vi "Sequence.Test.Engine.vi"(8 "error in (no error)":errorcluster, 11 "Data in":T1={"BeginTS"=timestamp(0 s since 1904-01-01), "EndTS"=timestamp(0 s since 1904-01-01), "State"=enum."Init", "Status.Work"=enum."-", "Status.Process"=enum."-", "Status.Home"=enum."-", "Status.Wabco"=enum."-", "Status.Client"=enum."-", "BreakReason"=enum."-", "BreakSource"=enum."-", "DoorLock"=FALSE, "Status.Prod"=[], "UserAction"={"Stop"=FALSE, "Pause"=FALSE, "Next"=FALSE}, "UserData"={"GuiMode"=enum."Process", "Test"={"IgnoreResults"=FALSE, "IgnoreImages"=FALSE, "ServiceMode"=FALSE}, "ContinueOrder"=FALSE}, "Error"={"status"=FALSE, "code"=0, "source"=""}, "Code"={"Ready"=FALSE, "DoubleOrder"=FALSE, "OrderDone"=FALSE, "AllowSingleSlot"=FALSE, "TunedA"=FALSE, "TunedB"=FALSE, "CheckDM"=FALSE, "ThresholdA"=0, "ThresholdB"=0, "Plate"=enum."Wabco", "ImgPath"=path "", "Variant"={"State"=enum."Init", "ImgPath"=path "", "WabcoPlate"="", "WabcoProduct"="", "ClientProduct"="", "ClientPlate"="", "TotalQuantity"=0, "OrderQuantity"=0, "Serial"=0, "Wabco"={"LaserJob"="", "AdditionalTxt"="037", "FactoryCode"="", "RevID"=0, "ForkID"=0, "FailuresLimit"=0, "GlobalCnt"=0, "Bank"=0, "SerialFormat"=enum."6 dig", "CoordA"={"X"=0.0, "Y"=0.0, "Angle"=0.0}, "CoordB"={"X"=0.0, "Y"=0.0, "Angle"=0.0}, "DMCconfig"=0}, "Client"={"LaserJob"="", "AdditionalTxt"="", "FactoryCode"="037", "RevID"=0, "ForkID"=0, "FailuresLimit"=0, "GlobalCnt"=0, "Bank"=0, "SerialFormat"=enum."6 dig", "CoordA"={"X"=0.0, "Y"=0.0, "Angle"=0.0}, "CoordB"={"X"=0.0, "Y"=0.0, "Angle"=0.0}, "DMCconfig"=0}}}, "Rotations"=0, "ProdIdx"=0, "ProdDone"=[], "PrintedSerials-Wabco"=[], "PrintedSerials-Client"=[], "Counters-Wabco"={"Expected"=0, "Done"=0, "OK"=0, "NOK"=0, "NOKlimit"=0, "Part"=0, "PartOK"=0}, "Counters-Client"={"Expected"=0, "Done"=0, "OK"=0, "NOK"=0, "NOKlimit"=0, "Part"=0, "PartOK"=0}}) -> (0 "error out":errorcluster, 3 "Data out":T1={"BeginTS"=timestamp(0 s since 1904-01-01), "EndTS"=timestamp(0 s since 1904-01-01), "State"=enum."Init", "Status.Work"=enum."-", "Status.Process"=enum."-", "Status.Home"=enum."-", "Status.Wabco"=enum."-", "Status.Client"=enum."-", "BreakReason"=enum."-", "BreakSource"=enum."-", "DoorLock"=FALSE, "Status.Prod"=[], "UserAction"={"Stop"=FALSE, "Pause"=FALSE, "Next"=FALSE}, "UserData"={"GuiMode"=enum."Process", "Test"={"IgnoreResults"=FALSE, "IgnoreImages"=FALSE, "ServiceMode"=FALSE}, "ContinueOrder"=FALSE}, "Error"={"status"=FALSE, "code"=0, "source"=""}, "Code"={"Ready"=FALSE, "DoubleOrder"=FALSE, "OrderDone"=FALSE, "AllowSingleSlot"=FALSE, "TunedA"=FALSE, "TunedB"=FALSE, "CheckDM"=FALSE, "ThresholdA"=0, "ThresholdB"=0, "Plate"=enum."Wabco", "ImgPath"=path "", "Variant"={"State"=enum."Init", "ImgPath"=path "", "WabcoPlate"="", "WabcoProduct"="", "ClientProduct"="", "ClientPlate"="", "TotalQuantity"=0, "OrderQuantity"=0, "Serial"=0, "Wabco"={"LaserJob"="", "AdditionalTxt"="037", "FactoryCode"="", "RevID"=0, "ForkID"=0, "FailuresLimit"=0, "GlobalCnt"=0, "Bank"=0, "SerialFormat"=enum."6 dig", "CoordA"={"X"=0.0, "Y"=0.0, "Angle"=0.0}, "CoordB"={"X"=0.0, "Y"=0.0, "Angle"=0.0}, "DMCconfig"=0}, "Client"={"LaserJob"="", "AdditionalTxt"="", "FactoryCode"="037", "RevID"=0, "ForkID"=0, "FailuresLimit"=0, "GlobalCnt"=0, "Bank"=0, "SerialFormat"=enum."6 dig", "CoordA"={"X"=0.0, "Y"=0.0, "Angle"=0.0}, "CoordB"={"X"=0.0, "Y"=0.0, "Angle"=0.0}, "DMCconfig"=0}}}, "Rotations"=0, "ProdIdx"=0, "ProdDone"=[], "PrintedSerials-Wabco"=[], "PrintedSerials-Client"=[], "Counters-Wabco"={"Expected"=0, "Done"=0, "OK"=0, "NOK"=0, "NOKlimit"=0, "Part"=0, "PartOK"=0}, "Counters-Client"={"Expected"=0, "Done"=0, "OK"=0, "NOK"=0, "NOKlimit"=0, "Part"=0, "PartOK"=0}})   [LabVIEW 2016]
uses:
  Sequence.Data.ctl
  Sequence.State.ctl
  Sequence.Step.Status.ctl
  Sequence.Test.BreakReason.ctl
  Sequence.Test.BreakSource.ctl
  Sequence.Test.Status.ctl
  Sequence.Slot.StatusData.ctl
  Sequence.Test.Unload.Status.ctl
  Sequence.Prod.StatusData.ctl
  Sequence.UserActions.ctl
  Sequence.UserData.ctl
  Sequence.MainMode.ctl
  Gui/MainGui.TestOptions.ctl
  Sequence.Code.Sets.ctl
  Sequence.PlateType.ctl
  Logger/Logger.Variant.Sets.ctl
  Station/Station.Changeover.State.vi
  Station/Station.Plate.Properties.ctl
  Sequence.Code.SerialFormat.ctl
  Drivers/V7310/LowLevel/V7310.Job.Sets.ctl
  Sequence.Counters.ctl
  Sequence.Global.vi
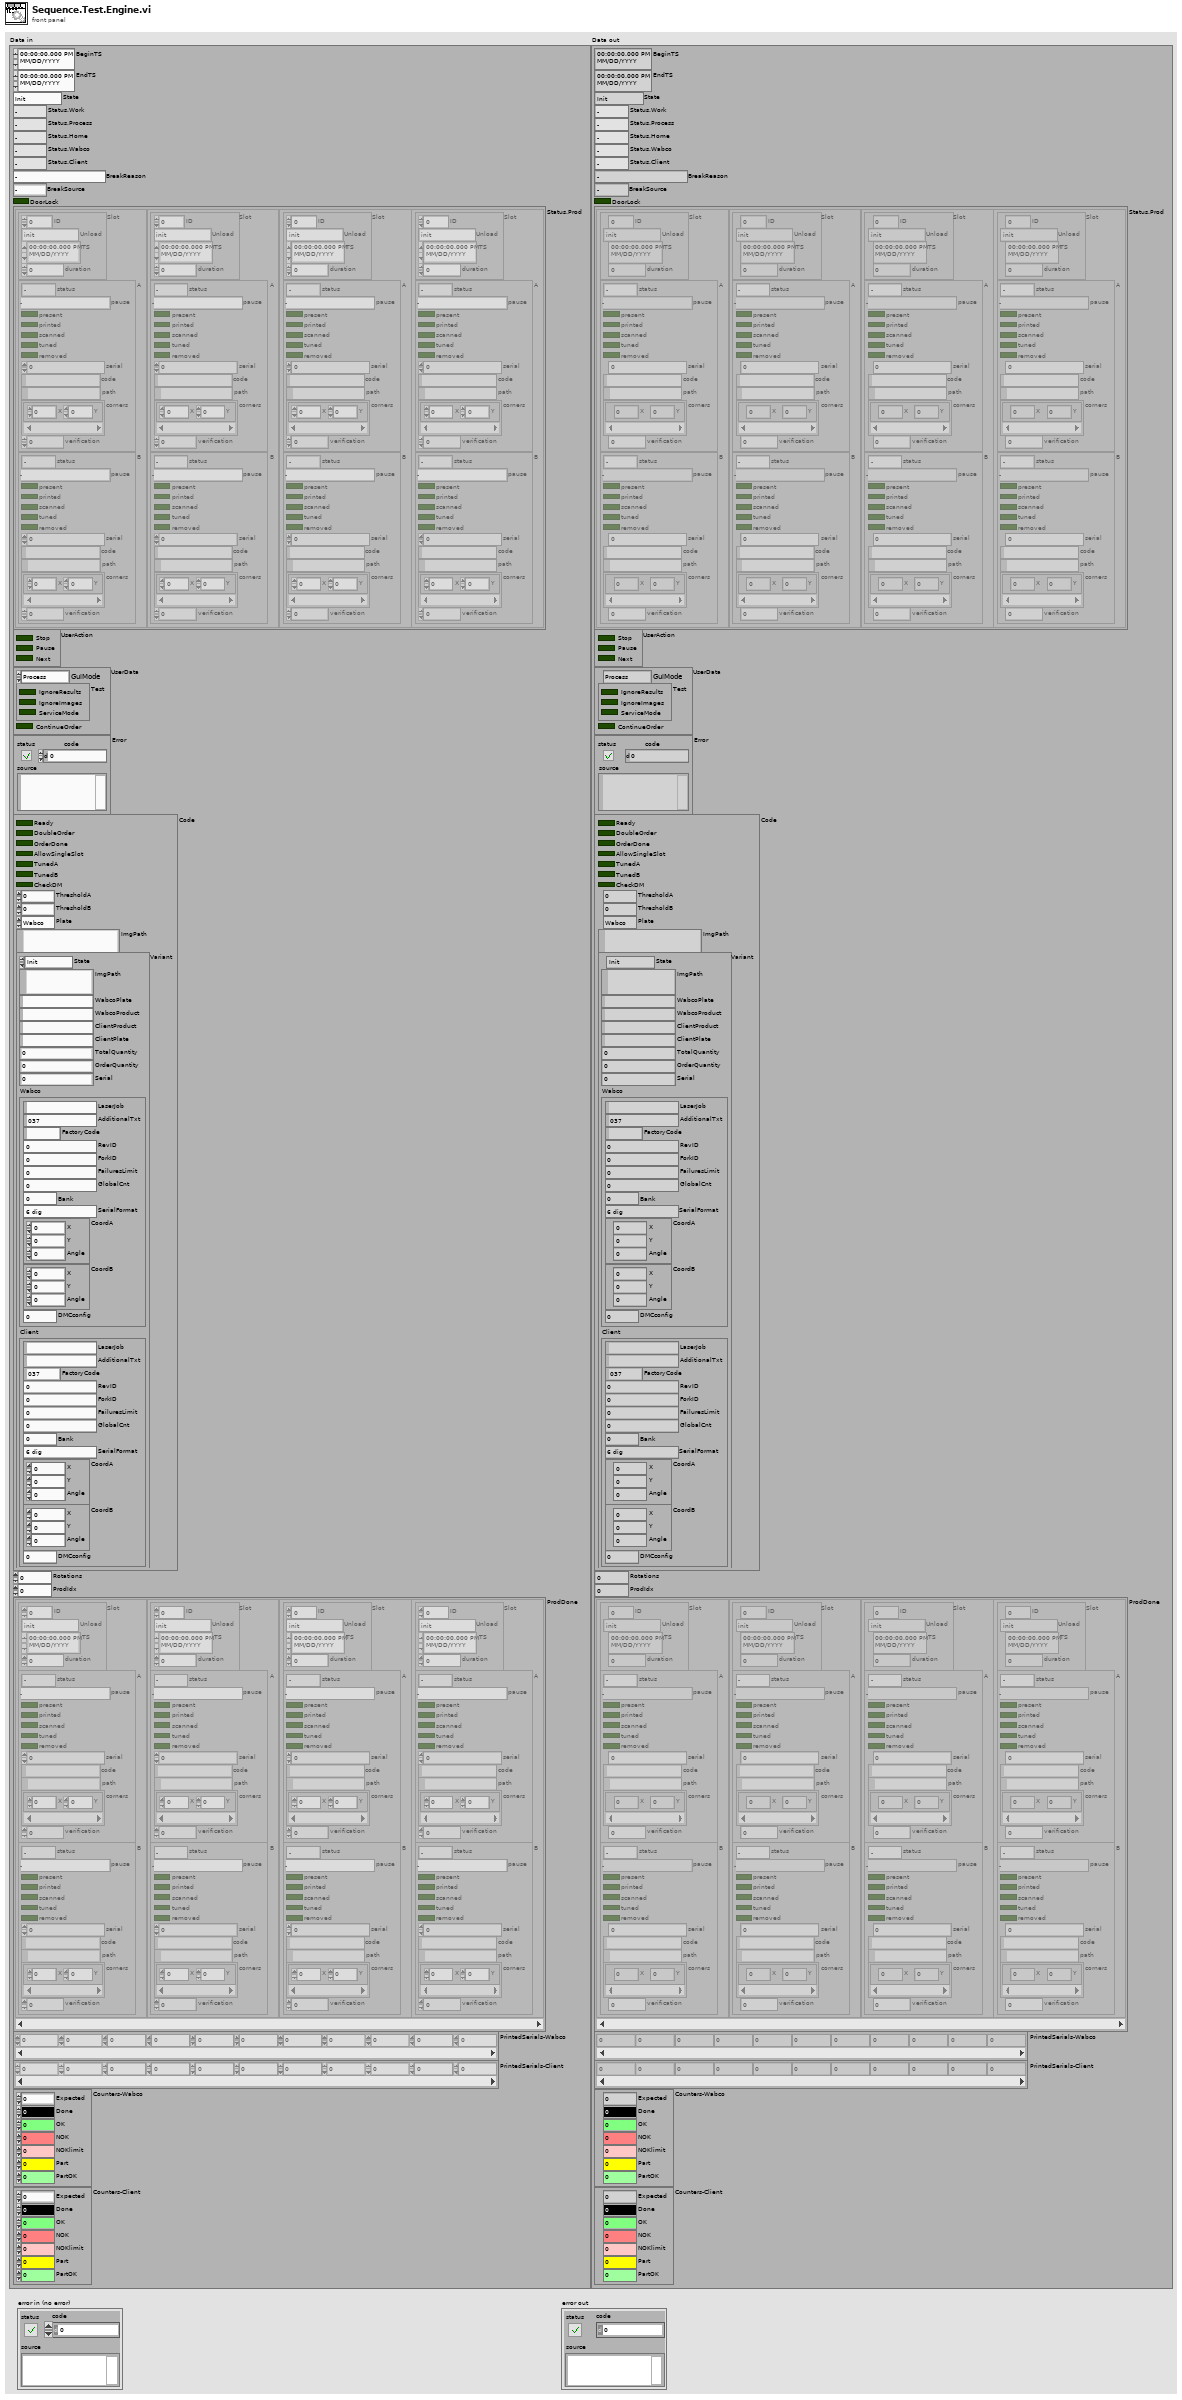
[diagram p1: front panel]
types:
  T1 = typedef "Sequence.Data.ctl" = cluster{"BeginTS":timestamp, "EndTS":timestamp, "State":T2, "Status.Work":T3, "Status.Process":T3, "Status.Home":T3, "Status.Wabco":T3, "Status.Client":T3, "BreakReason":T4, "BreakSource":T5, "DoorLock":bool, "Status.Prod":T6[], "UserAction":T10, "UserData":T11, "Error":errorcluster, "Code":T14, "Rotations":i32, "ProdIdx":i32, "ProdDone":T6[], "PrintedSerials-Wabco":i32[], "PrintedSerials-Client":i32[], "Counters-Wabco":T21, "Counters-Client":T21}
  T2 = typedef "Sequence.State.ctl" = enum16{"Init", "Idle", "Home", "Work", "Run", "Pause"}
  T3 = typedef "Sequence.Step.Status.ctl" = enum16{"-", "Pending", "Running", "Skipped", "Passed", "Failed", "Done", "Error", "Aborted", "Stopped"}
  T4 = typedef "Sequence.Test.BreakReason.ctl" = enum16{"-", "NOK container", "OK container", "Rev empty", "Rev missing", "Rev wrong", "Fork missing", "Fork wrong", "NOK limit", "Unload failure", "Single slot", "Part done", "Err: Prod move work", "Err: Prod move home", "Err: Prod lift work", "Err: Prod lift home", "Err: Prod Arm Work", "Err: Prod Arm NOK", "Err: Prod Arm OK", "Err: Prod NOK suck", "Err: Prod NOK drop", "Err: Prod OK missing", "Err: Prod OK suck", "Err: Prod OK drop"}
  T5 = typedef "Sequence.Test.BreakSource.ctl" = enum16{"-", "A", "B", "A/B"}
  T6 = typedef "Sequence.Test.Status.ctl" = cluster{"Slot":T7, "A":T9, "B":T9}
  T7 = typedef "Sequence.Slot.StatusData.ctl" = cluster{"ID":i32, "Unload":T8, "TS":timestamp, "duration":u32}
  T8 = typedef "Sequence.Test.Unload.Status.ctl" = enum16{"init", "check NOK", "check OK", "wait on NOK", "wait on OK", "wait on Unload", "done"}
  T9 = typedef "Sequence.Prod.StatusData.ctl" = cluster{"status":T3, "pause":T4, "present":bool, "printed":bool, "scanned":bool, "tuned":bool, "removed":bool, "serial":i32, "code":string, "path":path, "corners":cluster{"X":i32, "Y":i32}[], "verification":u8}
  T10 = typedef "Sequence.UserActions.ctl" = cluster{"Stop":bool, "Pause":bool, "Next":bool}
  T11 = typedef "Sequence.UserData.ctl" = cluster{"GuiMode":T12, "Test":T13, "ContinueOrder":bool}
  T12 = typedef "Sequence.MainMode.ctl" = enum16{"Process", "Base", "Order", "Manual", "Logs", "Results", "Stats", "DMC Config"}
  T13 = typedef "MainGui.TestOptions.ctl" = cluster{"IgnoreResults":bool, "IgnoreImages":bool, "ServiceMode":bool}
  T14 = typedef "Sequence.Code.Sets.ctl" = cluster{"Ready":bool, "DoubleOrder":bool, "OrderDone":bool, "AllowSingleSlot":bool, "TunedA":bool, "TunedB":bool, "CheckDM":bool, "ThresholdA":u8, "ThresholdB":u8, "Plate":T15, "ImgPath":path, "Variant":T16}
  T15 = typedef "Sequence.PlateType.ctl" = enum16{"Wabco", "Client"}
  T16 = typedef "Logger.Variant.Sets.ctl" = cluster{"State":T17, "ImgPath":path, "WabcoPlate":string, "WabcoProduct":string, "ClientProduct":string, "ClientPlate":string, "TotalQuantity":u16, "OrderQuantity":u16, "Serial":i32, "Wabco":T18, "Client":T18}
  T17 = typedef "Station.Changeover.State.vi" = enum16{"Init", "Scaning", "NOK", "Wait for ack", "Ready"}
  T18 = typedef "Station.Plate.Properties.ctl" = cluster{"LaserJob":string, "AdditionalTxt":string, "FactoryCode":string, "RevID":u8, "ForkID":u8, "FailuresLimit":u16, "GlobalCnt":i32, "Bank":u8, "SerialFormat":T19, "CoordA":T20, "CoordB":T20, "DMCconfig":i32}
  T19 = typedef "Sequence.Code.SerialFormat.ctl" = enum8{"", "6 dig", "7 dig"}
  T20 = typedef "V7310.Job.Sets.ctl" = cluster{"X":dbl, "Y":dbl, "Angle":dbl}
  T21 = typedef "Sequence.Counters.ctl" = cluster{"Expected":u16, "Done":u16, "OK":u16, "NOK":u16, "NOKlimit":u16, "Part":u16, "PartOK":u16}
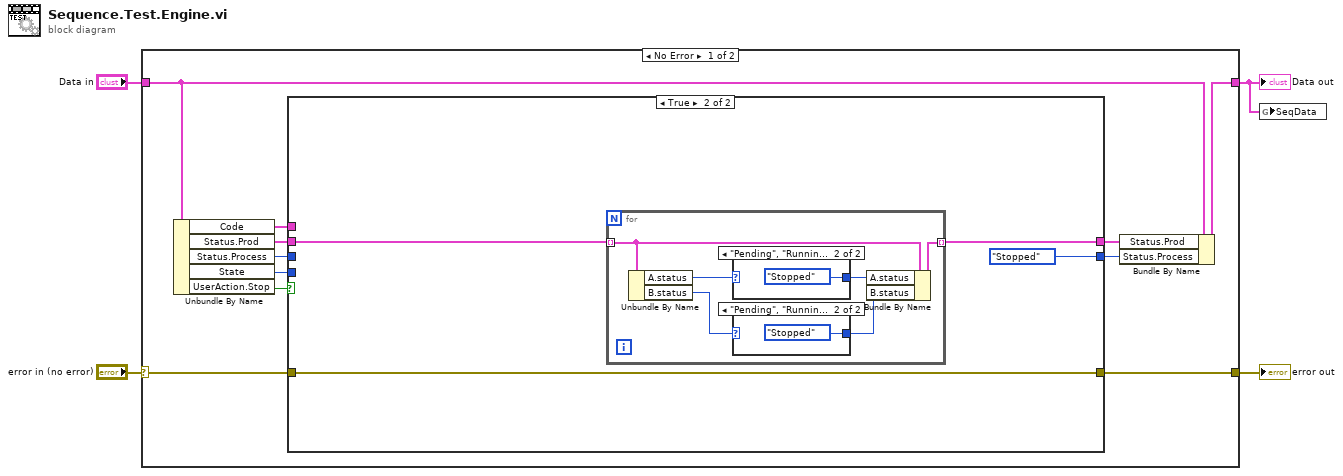
[diagram p0: block diagram]
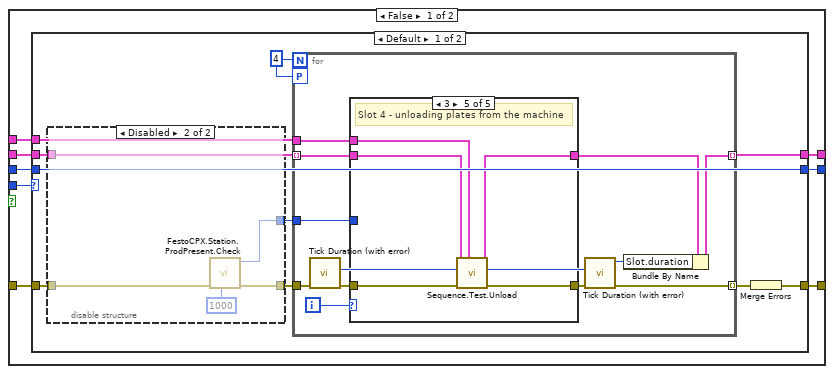
[diagram p2: hidden frame]
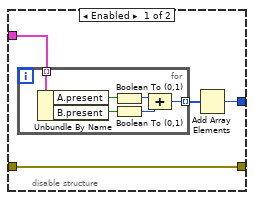
[diagram p3: hidden frame]
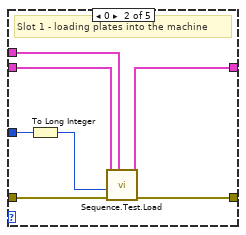
[diagram p5: hidden frame]
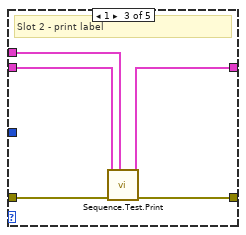
[diagram p6: hidden frame]
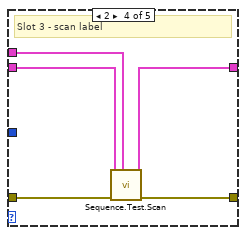
[diagram p7: hidden frame]
diagram:
  n1 = case shown="No Error" "error in (no error)" {
    selector: "error in (no error)" -> [w5 w101]
    tunnel: [w12 w101] -> w4
    tunnel: [w14 w102] -> w1
    tunnel: "Data in" -> [w15 w102]
    frame No Error {
      n2 = Unbundle By Name(w15) -> ("Code"=w11:T14, "Status.Prod"=w6:T6[], "Status.Process"=w10:T3, "State"=w8:T2, "UserAction.Stop"=w7:bool)
      n3 = case shown="True" w7 {
        tunnel: w6 -> [w23 w90]
        tunnel: [w22 w89] -> w13
        tunnel: [w21 w87] -> w12
        tunnel: w11 -> [w20 _]
        tunnel: w5 -> [w19 w87]
        tunnel: w10 -> [w18 _]
        tunnel: [w17 Sequence.Step.Status."Stopped" ("A.status")] -> w9
        tunnel: w8 -> [w16 _]
        frame False {
          n4 = case shown="Default" w16 {
            tunnel: w23 -> [w27 w86]
            tunnel: [w33 w86] -> w22
            tunnel: [w32 w84] -> w21
            tunnel: w20 -> [w31 _]
            tunnel: w19 -> [w26 w84]
            tunnel: w18 -> [w30 w85]
            tunnel: [w30 w85] -> w17
            frame Default {
              w24 = 4
              n5 = disable-structure shown="Disabled" {
                disable-tunnel: [w36 w46] -> w28
                disable-tunnel: w27 -> [w35 _]
                disable-tunnel: w26 -> [w34 w45]
                disable-tunnel: [w34 w47] -> w25
                frame Enabled {
                  n6 = for {
                    tunnel: w35 -> [w43] mode=indexing
                    tunnel: [w38] -> w37 mode=indexing
                    n7 = Unbundle By Name(w43) -> ("A.present"=w41:bool, "B.present"=w42:bool)
                    n8 = Boolean To (0,1)(Boolean=w41) -> (0, 1=w40:i16)
                    n9 = Boolean To (0,1)(Boolean=w42) -> (0, 1=w39:i16)
                    n10 = Compound Arithmetic op=ADD(w40, w39) -> (w38:i16)
                  }
                  n11 = Add Array Elements(numeric array=w37) -> (sum=w36:i16)
                }
                frame Disabled {
                  n12 = call "FestoCPX.Station.ProdPresent.Check.vi"("Stab Counter (0)"=u32 1000 ("Max Stab time [ms] (0)"), "error in"=w45) -> ("error out"=w47:errorcluster, "#products in the machine"=w46:i32)  [unwired: 4 in, 4 out]
                }
              }
              n13 = for {
                N: w24 -> [_]
                tunnel: w25 -> [w56]
                workers-P: w24 -> [_]
                tunnel: w27 -> [w58] mode=indexing
                tunnel: [w51] -> w29 mode=indexing
                tunnel: [w50] -> w33 mode=indexing
                tunnel: w31 -> [w57]
                tunnel: w28 -> [w49]
                i -> [w59]
                n14 = call "Tick Duration (with error).vi"("error in (no error)"=w56) -> ("error out"=w55:errorcluster, "tick count after [ms]"=w53:u32)  [unwired: 8 in, 1 out]
                n15 = case shown="3" w59 {
                  tunnel: w55 -> [w61 w68 w73 w78 w82]
                  tunnel: [w61 w65 w70 w74 w81] -> w54
                  tunnel: w58 -> [w60 w67 w72 w77 w83]
                  tunnel: [w60 w66 w71 w76 w79] -> w52
                  tunnel: w57 -> [_ w64 w69 w75 w80]
                  tunnel: w49 -> [_ w63 _ _ _]
                  frame Default {
                  }
                  frame 0 {
                    # "Slot 1 - loading plates into the machine"
                    n16 = To Long Integer(number=w63) -> (32bit integer=w62:i32)
                    n17 = call "Sequence.Test.Load.vi"("Code in"=w64, "error in"=w68, "#products in the machine"=w62, "Data in"=w67) -> ("error out"=w65:errorcluster, "Data out"=w66:T6)  [unwired: 6 in]
                  }
                  frame 1 {
                    # "Slot 2 - print label"
                    n18 = call "Sequence.Test.Print.vi"("Code in"=w69, "error in"=w73, "Data in"=w72) -> ("error out"=w70:errorcluster, "Data out"=w71:T6)  [unwired: 7 in]
                  }
                  frame 2 {
                    # "Slot 3 - scan label"
                    n19 = call "Sequence.Test.Scan.vi"("Code"=w75, "error in"=w78, "Data in"=w77) -> ("error out"=w74:errorcluster, "Data out"=w76:T6)  [unwired: 7 in]
                  }
                  frame 3 {
                    # "Slot 4 - unloading plates from the machine"
                    n20 = call "Sequence.Test.Unload.vi"("Code in"=w80, "error in"=w82, "Data in"=w83) -> ("error out"=w81:errorcluster, "Data out"=w79:T6)  [unwired: 7 in]
                  }
                }
                n21 = call "Tick Duration (with error).vi"("error in (no error)"=w54, "tick count before"=w53) -> ("error out"=w51:errorcluster, "duration [ms]"=w48:u32)  [unwired: 7 in, 1 out]
                n22 = Bundle By Name(cluster=w52, "Slot.duration"=w48) -> (w50:T6)
              }
              n23 = Merge Errors(w29) -> (w32:errorcluster)
            }
            frame "Pause" {
            }
          }
        }
        frame True {
          n24 = for {
            tunnel: w90 -> [w95] mode=indexing
            tunnel: [w96] -> w89 mode=indexing
            n25 = Unbundle By Name(w95) -> ("A.status"=w94:T3, "B.status"=w91:T3)
            n26 = case shown="\"Pending\", \"Running\"" w94 {
              selector: w94 -> [w99 _]
              tunnel: [w99 Sequence.Step.Status."Stopped" ("A.status")] -> w93
              frame Default {
              }
              frame "Pending", "Running" {
              }
            }
            n27 = case shown="\"Pending\", \"Running\"" w91 {
              selector: w91 -> [w97 _]
              tunnel: [w97 Sequence.Step.Status."Stopped" ("A.status")] -> w92
              frame Default {
              }
              frame "Pending", "Running" {
              }
            }
            n28 = Bundle By Name(cluster=w95, "A.status"=w93, "B.status"=w92) -> (w96:T6)
          }
        }
      }
      n29 = Bundle By Name(cluster=w15, "Status.Prod"=w13, "Status.Process"=w9) -> (w14:T1)
    }
    frame Error {
    }
  }
  "error out" <- w4
  "Data out" <- w1
  n30 = global write "Sequence.Global.vi" "SeqData"(w1) -> ()
